vi "EMD8216 password change.vi"(9 "Password":string, 10 "Oldpassword":string, 11 "CardID":u32) -> (3 "error_code":u32)   [LabVIEW 2009, in "EMD8216_64.lvlib"]
doc: "EMD8216Status EMD8216_password_change(u32 CardID,u8 Oldpassword[8],u8 Password[8]);"
uses:
  EMD8216_64.lvlib
  <userlib>/EMD8216_64/EMD8216_64.dll
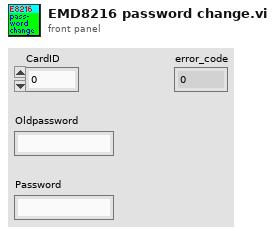
[diagram p1: front panel]
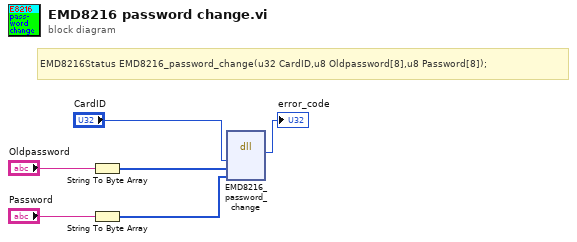
[diagram p0: block diagram]
diagram:
  # "EMD8216Status EMD8216_password_change(u32 CardID,u8 Oldpassword[8],u8 Password[8]);"
  n1 = String To Byte Array(string="Oldpassword") -> (unsigned byte array=w1:u8[])
  n2 = String To Byte Array(string="Password") -> (unsigned byte array=w2:u8[])
  n3 = dll-call lib="C:/Program Files/National Instruments/LabVIEW 2017/user.lib/EMD8216_64/EMD8216_64.*" fn="EMD8216_password_change"("CardID"="CardID", "Oldpassword"=w1, "Password"=w2) -> ("return type"=→"error_code":u32)  [unwired: 6 in, 2 out]
